vi "减去左移100.vi"(0 "输入字符串":string="AT\u0007è\f\b\u0005p\u0000\u0000\u0001\u0000\u0000\u0000\r\n") -> (1 "结果字符串":string, 2 "替换子字符串":string, 3 "16进制转换":string)   [LabVIEW 2023]
panel:
  out "二进制字节长度":i32
  out "十进制数":i32
  out "截取包含电机canid的字符串":string
  out "该删者":string
  out "删除左移100后":string
  out "转成二进制":string
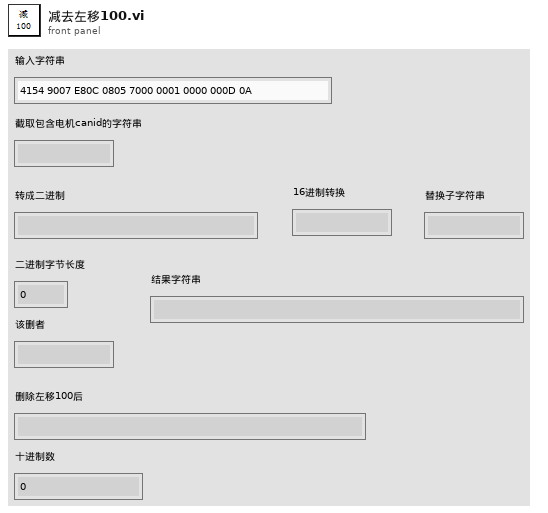
[diagram p1: front panel]
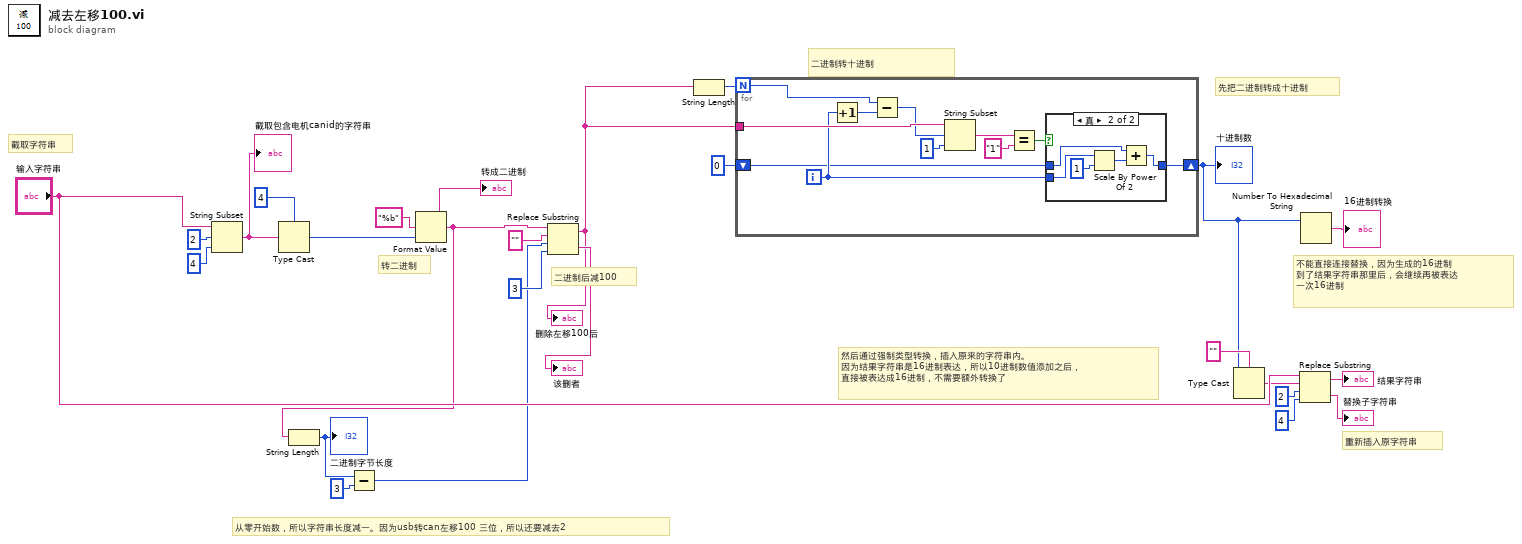
[diagram p0: block diagram]
diagram:
  # "然后通过强制类型转换，插入原来的字符串内。\n因为结果字符串是16进制表达，所以10进制数值添加之后，\n直接被表达成16进制，不需要额外转换了"
  # "先把二进制转成十进制"
  # "不能直接连接替换，因为生成的16进制\n到了结果字符串那里后，会继续再被表达\n一次16进制"
  # "从零开始数，所以字符串长度减一。因为usb转can左移100 三位，所以还要减去2"
  # "重新插入原字符串"
  # "二进制后减100"
  # "转二进制"
  # "截取字符串"
  # "二进制转十进制"
  n1 = String Subset(string="输入字符串", offset (0)=2 ("偏移量(0)"), length (rest)=4 ("长度（剩余）")) -> (substring=w22:string)
  "截取包含电机canid的字符串" <- w22
  n2 = Type Cast(type=4 ("长度（剩余）"), x=w22) -> (*(type *) &x=w20:i32)
  n3 = Format Value(format string="%b" ("格式字符串"), value (0)=w20) -> (output string=w8:string)  [unwired: 1 in]
  "转成二进制" <- w8
  n4 = String Length(string=w8) -> (length=w7:i32)
  "二进制字节长度" <- w7
  n5 = Subtract(x=w7, y=3) -> (x-y=w5:i32)
  n6 = Replace Substring(2:3 ("长度（子字符串长度）"), 3:w5, 4:"" ("子字符串(\"\")"), 5:w8) -> (0:→"该删者":string, 1:w14:string)
  "删除左移100后" <- w14
  n7 = String Length(string=w14) -> (length=w16:i32)
  n8 = for {
    N: w16 -> [w34]
    tunnel: w14 -> [w36]
    shift-right: [w26] -> w1
    shift-left: 0 ("长度（剩余）") -> [w27]
    i -> [w28]
    n9 = Increment(x=w28) -> (x+1=w32:i32)
    n10 = Subtract(x=w34, y=w32) -> (x-y=w33:i32)
    n11 = String Subset(string=w36, offset (0)=w33, length (rest)=1 ("长度（剩余）")) -> (substring=w31:string)
    n12 = Equal?(x=w31, y="1") -> (x = y?=w29:bool)
    n13 = case shown="真" w29 {
      tunnel: w28 -> [_ w42]
      tunnel: w27 -> [w37 w41]
      tunnel: [w37 w39] -> w26
      frame False {
      }
      frame True {
        n14 = Scale By Power Of 2(n=w42, x=1) -> (x*2^n=w38:i32)
        n15 = Add(x=w41, y=w38) -> (x+y=w39:i32)
      }
    }
  }
  "十进制数" <- w1
  n16 = Type Cast(type="", x=w1) -> (*(type *) &x=w2:string)
  n17 = Replace Substring(2:4 ("长度（子字符串长度）"), 3:2 ("偏移量(0)"), 4:w2, 5:"输入字符串") -> (0:→"替换子字符串":string, 1:→"结果字符串":string)
  n18 = Number To Hexadecimal String(2:w1) -> (0:→"16进制转换":string)  [unwired: 1 in]
